vi "Run Status Code to String.vi"(10 "Code":u16 caption="代码") -> (2 "Info String":string caption="信息")   [LabVIEW 2023, in "Longer Pump dLSP501 Series.lvlib"]
uses:
  <instrlib>/Longer Pump dLSP501 Modbus RTU Series/Longer Pump dLSP501 Series.lvlib
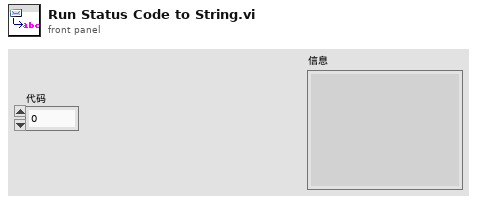
[diagram p1: front panel]
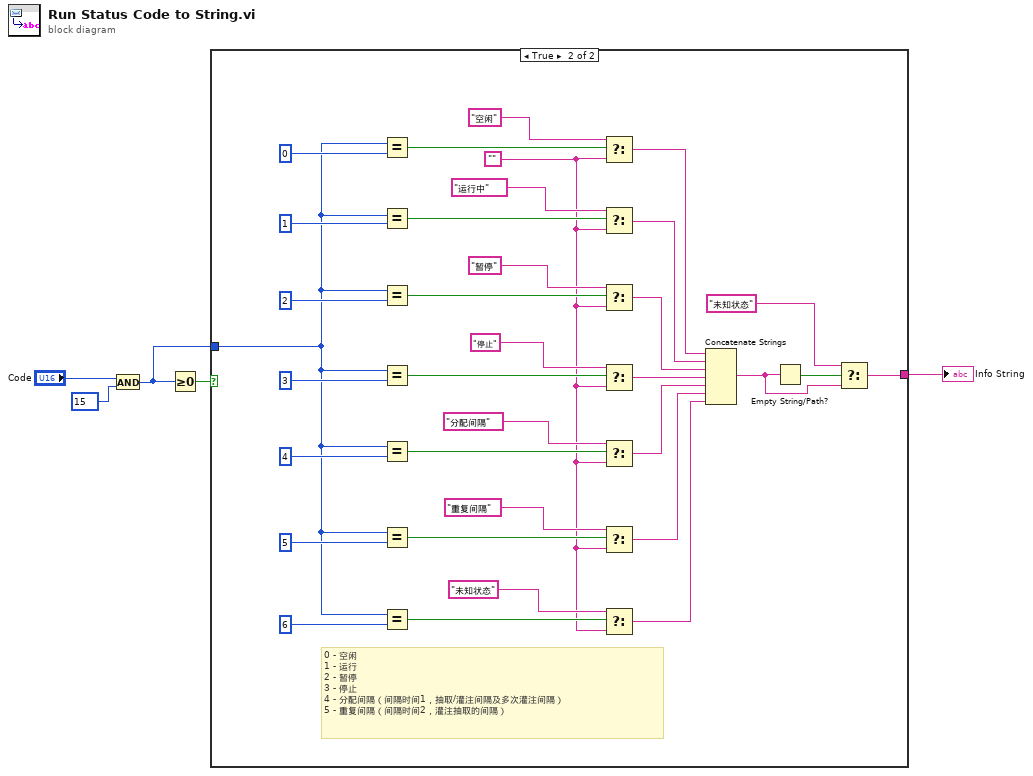
[diagram p0: block diagram]
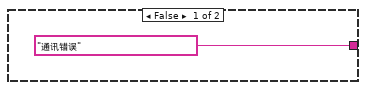
[diagram p2: hidden frame]
diagram:
  n1 = And(x="Code", y=u16 15 ("x")) -> (x .and. y?=w2:u16)
  n2 = Greater Or Equal To 0?(x=w2) -> (x >= 0?=w5:bool)
  n3 = case shown="True" w5 {
    tunnel: ["通讯错误" ("Status 2") w29] -> w4
    tunnel: w2 -> [_ w17]
    frame False {
    }
    frame True {
      w7 = ""
      # "0 - 空闲\n1 - 运行\n2 - 暂停  \n3 - 停止  \n4 - 分配间隔（间隔时间1，抽取/灌注间隔及多次灌注间隔）  \n5 - 重复间隔（间隔时间2，灌注抽取的间隔）"
      n4 = Equal?(x=w17, y=u32 0) -> (x = y?=w40:bool)
      n5 = Equal?(x=w17, y=u32 1) -> (x = y?=w39:bool)
      n6 = Equal?(x=w17, y=u32 2) -> (x = y?=w38:bool)
      n7 = Equal?(x=w17, y=u32 3) -> (x = y?=w37:bool)
      n8 = Equal?(x=w17, y=u32 4) -> (x = y?=w36:bool)
      n9 = Equal?(x=w17, y=u32 5) -> (x = y?=w32:bool)
      n10 = Equal?(x=w17, y=u32 6) -> (x = y?=w26:bool)
      n11 = Select(t="空闲" ("Status 2"), s=w40, f=w7) -> (s? t:f=w16:string)
      n12 = Select(t="运行中" ("Status 2"), s=w39, f=w7) -> (s? t:f=w8:string)
      n13 = Select(t="暂停" ("Status 2"), s=w38, f=w7) -> (s? t:f=w35:string)
      n14 = Select(t="停止" ("Status 2"), s=w37, f=w7) -> (s? t:f=w33:string)
      n15 = Select(t="分配间隔" ("Status 2"), s=w36, f=w7) -> (s? t:f=w34:string)
      n16 = Select(t="重复间隔" ("Status 2"), s=w32, f=w7) -> (s? t:f=w31:string)
      n17 = Select(t="未知状态" ("Status 2"), s=w26, f=w7) -> (s? t:f=w25:string)
      n18 = Concatenate Strings(w16, w8, w35, w33, w34, w31, w25) -> (w30:string)
      n19 = Empty String/Path?(string/path=w30) -> (empty?=w28:bool)
      n20 = Select(t="未知状态", s=w28, f=w30) -> (s? t:f=w29:string)
    }
  }
  "Info String" <- w4
